vi "GPIO Event.vi"() -> ()   [LabVIEW 2017]
uses:
  IMAQCV/GPIO/GPIO Pins.ctl
  IMAQCV/PIIO.lvlib
panel:
  in  "stop":bool
  out "DI-CH4":bool
  out "DI-CH3":bool
  out "DI-CH2":bool
  out "DI-CH1":bool
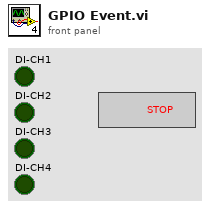
[diagram p1: front panel]
types:
  T1 = typedef "PIIO.lvlib/GPIO Pins.ctl" = u8
  T2 = cluster{"GPIO":T1[], "MODE":enum8{"INPUT", "OUTPUT"}[]}
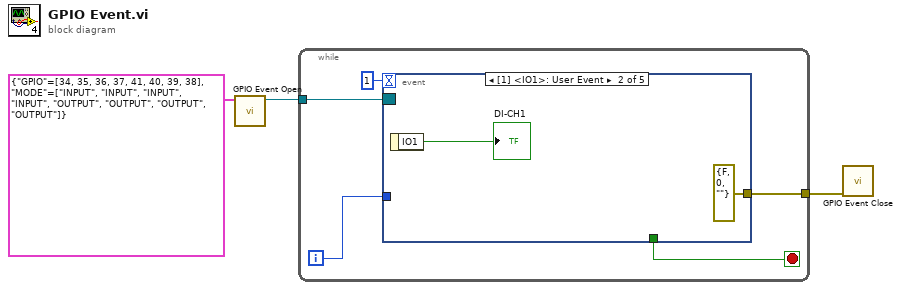
[diagram p0: block diagram]
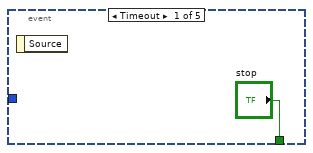
[diagram p2: hidden frame]
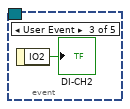
[diagram p3: hidden frame]
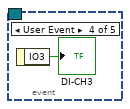
[diagram p4: hidden frame]
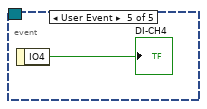
[diagram p5: hidden frame]
diagram:
  n1 = call "GPIO Event Open.vi"("GPIO"=T2 {"GPIO"=[34, 35, 36, 37, 41, 40, 39, 38], "MODE"=[enum."INPUT", enum."INPUT", enum."INPUT", enum."INPUT", enum."OUTPUT", enum."OUTPUT", enum."OUTPUT", enum."OUTPUT"]}) -> ("Event Registration Refnum"=w3:refnum<event-registration>)  [unwired: 9 in, 1 out]
  n2 = while {
    tunnel: w3 -> [w5]
    tunnel: [w4] -> w2
    i -> [w8]
    stop <- w7 stop-if-true
    n3 = event shown="[1] <IO1>: User Event" {
      selector: w5 -> [_ _ _ _ _]
      dyn-events: _ -> [_ _ _ _ _]
      timeout: 1 -> [_ _ _ _ _]
      tunnel: w8 -> [_ _ _ _ _]
      tunnel: ["stop" _ _ _ _] -> w7
      tunnel: [_ errorcluster {"status"=FALSE, "code"=0, "source"=""} ("error out") _ _ _] -> w4
      event Timeout {
        n4 = event-data() -> ()  [unwired: 1 in, 1 out]
      }
      event User Event {
        n5 = event-data() -> ("IO1"=→"DI-CH1":bool)  [unwired: 1 in]
      }
      event User Event {
        n6 = event-data() -> ("IO2"=→"DI-CH2":bool)  [unwired: 1 in]
      }
      event User Event {
        n7 = event-data() -> ("IO3"=→"DI-CH3":bool)  [unwired: 1 in]
      }
      event User Event {
        n8 = event-data() -> ("IO4"=→"DI-CH4":bool)  [unwired: 1 in]
      }
    }
  }
  n9 = call "GPIO Event Close.vi"("error in (no error)"=w2) -> ()  [unwired: 10 in, 1 out]
